vi "Custom VISA Enumerate.vi"(5 "Force refresh? (False)":bool, 7 "Interface filter (all)":T1={"GPIB"=TRUE, "Serial"=TRUE, "TCP"=TRUE, "USB"=TRUE}, 8 "error in (no error)":errorcluster, 9 "Last VISA address (empty)":refnum<visa-resource-name>, 10 "Last VISA selector Value (none)":u16=65535, 11 "VISA menu ref":refnum<vi>) -> (0 "error out":errorcluster, 2 "VISA list":string[](array[string]), 3 "Selected VISA address":refnum<visa-resource-name>)   [LabVIEW 2020, in "Get COM Descriptor.lvlib"]
doc: "When Ring.Text = \"Refresh\", Enumerates VISA devices using interface filter options, fills Ring control with the list. It appends COM port descriptors to COM port names. Call this in Ring Value Change event. You can also force re-enumeration despite Ring.Text value. In case of Refresh, it tries to select Last VISA address item if provided or Last VISA selector value if provided.\nIt outputs selected VISA address. \n\nDetails: https://github.com/smaslan/get-com-descriptor"
uses:
  Get COM Descriptor.lvlib
  Custom VISA Filters.ctl
  fe2b3fdb-a69f-4816-a13d-02b51eb7bdf9.vi
  0cf15640-2a7e-453d-a7d5-3e9773abd412.vi
  <vilib>/Comparison/Equal/Equal Functor/Equal Functor.lvclass
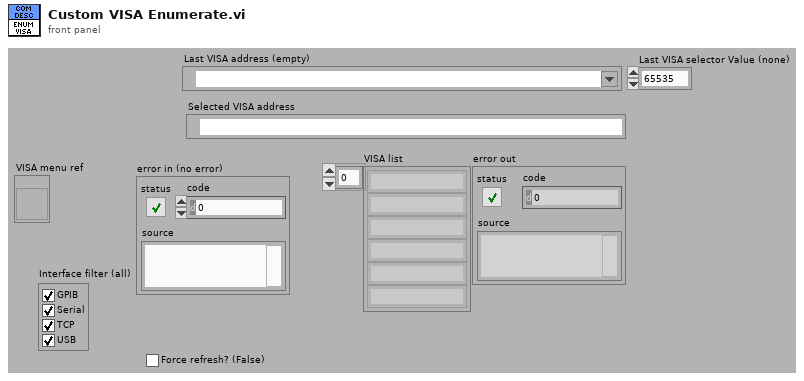
[diagram p1: front panel]
types:
  T1 = typedef "Get COM Descriptor.lvlib/Custom VISA Filters.ctl" = cluster{"GPIB":bool, "Serial":bool, "TCP":bool, "USB":bool}
  T2 = typedef "Get COM Descriptor.lvlib/COM port.ctl" = cluster{"port":string, "descriptor":string}
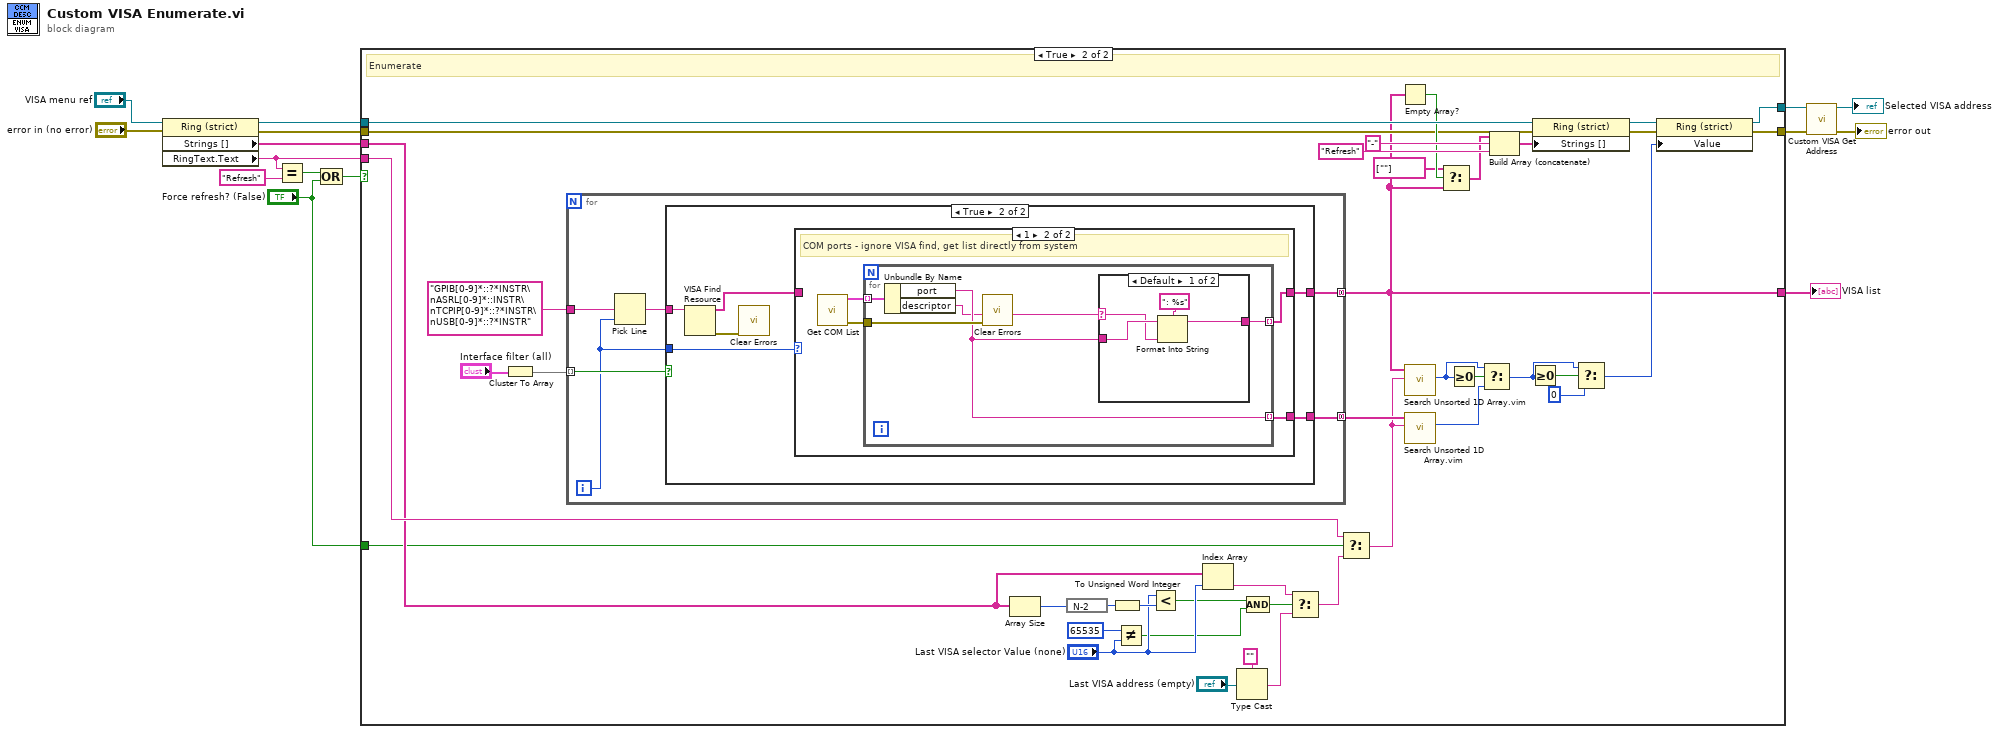
[diagram p0: block diagram]
diagram:
  n1 = property class="Ring (strict)"(reference="VISA menu ref", error in="error in (no error)") -> (reference out=w14:refnum<vi>, error out=w13:errorcluster, "Strings []"=w1:string[], "RingText.Text"=w8:string)
  n2 = Equal?(x=w8, y="Refresh") -> (x = y?=w10:bool)
  n3 = Compound Arithmetic op=OR(w10, "Force refresh? (False)") -> (w9:bool)
  n4 = case shown="True" w9 {
    tunnel: w14 -> [w16 w52]
    tunnel: w13 -> [w17 w46]
    tunnel: [w17 w45] -> w7
    tunnel: w8 -> [_ w33]
    tunnel: [w16 w36] -> w5
    tunnel: [_ w35] -> w3
    tunnel: "Force refresh? (False)" -> [_ w18]
    tunnel: w1 -> [_ w26]
    frame False {
    }
    frame True {
      # "Enumerate"
      n5 = Cluster To Array(cluster="Interface filter (all)") -> (array=w57:bool[])
      n6 = for {
        tunnel: w57 -> [w63] mode=indexing
        tunnel: "GPIB[0-9]*::?*INSTR\nASRL[0-9]*::INSTR\nTCPIP[0-9]*::?*INSTR\nUSB[0-9]*::?*INSTR" -> [w64]
        tunnel: [w61] -> w35 mode=concatenating
        tunnel: [w59] -> w44 mode=concatenating
        i -> [w60]
        n7 = Pick Line(multi-line string=w64, line index=w60) -> (output string=w62:string)  [unwired: 1 in]
        n8 = case shown="True" w63 {
          tunnel: w62 -> [_ w70]
          tunnel: [_ w66] -> w61
          tunnel: w60 -> [_ w68]
          tunnel: [_ w65] -> w59
          frame False {
          }
          frame True {
            n9 = VISA Find Resource(11:w70) -> (0:w69:errorcluster, 3:w67:string[])  [unwired: 2 in, 1 out]
            n10 = call <vilib>:"Clear Errors.vi"("error in (no error)"=w69) -> ()  [unwired: 5 in, 2 out]
            n11 = case shown="1" w68 {
              tunnel: w67 -> [w71 _]
              tunnel: [w71 w75] -> w66
              tunnel: [w71 w74] -> w65
              frame Default {
              }
              frame 1 {
                # "COM ports - ignore VISA find, get list directly from system"
                n12 = call "Get COM List.vi"() -> ("error out"=w73:errorcluster, "COM list"=w72:T2[])  [unwired: 8 in, 2 out]
                n13 = for {
                  tunnel: [w80] -> w75 mode=indexing
                  tunnel: [w77] -> w74 mode=indexing
                  tunnel: w73 -> [w78]
                  tunnel: w72 -> [w79] mode=indexing
                  n14 = Unbundle By Name(w79) -> ("port"=w77:string, "descriptor"=w76:string)
                  n15 = call <vilib>:"Clear Errors.vi"("error in (no error)"=w78) -> ()  [unwired: 5 in, 2 out]
                  n16 = case shown="Default" w76 {
                    selector: w76 -> [w81 _]
                    tunnel: w77 -> [w82 w85]
                    tunnel: [w83 w85] -> w80
                    frame Default {
                      n17 = Format Into String(format string=": %s", initial string=w82, w81) -> (resulting string=w83:string)  [unwired: 1 in, 1 out]
                    }
                    frame "" {
                    }
                  }
                }
              }
            }
          }
        }
      }
      n18 = Array Size(array=w26) -> (size(s)=w29:i32)
      n19 = expression code="N-2"(w29) -> (w28:i32)
      n20 = To Unsigned Word Integer(number=w28) -> (unsigned 16bit integer=w27:u16)
      n21 = Not Equal?(x=u16 65535, y="Last VISA selector Value (none)") -> (x != y?=w23:bool)
      n22 = Less?(x="Last VISA selector Value (none)", y=w27) -> (x < y?=w24:bool)
      n23 = Index Array(array=w26, index="Last VISA selector Value (none)") -> (element=w21:string)
      n24 = Type Cast(type="", x="Last VISA address (empty)") -> (*(type *) &x=w20:string)
      n25 = Compound Arithmetic op=AND(w24, w23) -> (w22:bool)
      n26 = Select(t=w21, s=w22, f=w20) -> (s? t:f=w19:string)
      n27 = Select(t=w33, s=w18, f=w19) -> (s? t:f=w34:string)
      n28 = Empty Array?(array=w35) -> (empty?=w51:bool)
      n29 = call "Search Unsorted 1D Array.vim"("element"=w34, "unsorted 1D array"=w35) -> ("index of element"=w42:i32)  [unwired: 9 in]
      n30 = call "Search Unsorted 1D Array.vim"("element"=w34, "unsorted 1D array"=w44) -> ("index of element"=w41:i32)  [unwired: 9 in]
      n31 = Select(t=string[] [""], s=w51, f=w35) -> (s? t:f=w50:string[])
      n32 = Greater Or Equal To 0?(x=w42) -> (x >= 0?=w43:bool)
      n33 = Select(t=w42, s=w43, f=w41) -> (s? t:f=w39:i32)
      n34 = Build Array (concatenate)(w50, "-" ("element"), "Refresh") -> (w53:string[])
      n35 = Greater Or Equal To 0?(x=w39) -> (x >= 0?=w40:bool)
      n36 = property class="Ring (strict)"(reference=w52, error in=w46, "Strings []"=w53) -> (reference out=w47:refnum<vi>, error out=w48:errorcluster)
      n37 = Select(t=w39, s=w40, f=0) -> (s? t:f=w37:i32)
      n38 = property class="Ring (strict)"(reference=w47, error in=w48, "Value"=w37) -> (reference out=w36:refnum<vi>, error out=w45:errorcluster)
    }
  }
  "VISA list" <- w3
  n39 = call "Custom VISA Get Address.vi"("error in (no error)"=w7, "VISA menu ref"=w5) -> ("error out"=→"error out":errorcluster, "VISA address"=→"Selected VISA address":refnum<visa-resource-name>)  [unwired: 8 in]
